vi "parseCameraData.vi"() -> (3 "TargetInfoOut":T1)   [LabVIEW 2012]
uses:
  2013NewCan/Robot Global Data.vi
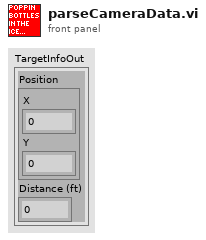
[diagram p1: front panel]
types:
  T1 = cluster{"Position":cluster{"X":dbl, "Y":dbl}, "Distance (ft)":dbl}
  T2 = cluster{"Position":cluster{"X":dbl, "Y":dbl}, "Distance (ft)":dbl}[]
  T3 = cluster{"Target Info[0]":cluster{"Position":cluster{"X":dbl, "Y":dbl}, "Distance (ft)":dbl}, "Target Info[1]":cluster{"Position":cluster{"X":dbl, "Y":dbl}, "Distance (ft)":dbl}, "Target Info[2]":cluster{"Position":cluster{"X":dbl, "Y":dbl}, "Distance (ft)":dbl}, "Target Info[3]":cluster{"Position":cluster{"X":dbl, "Y":dbl}, "Distance (ft)":dbl}, "Target Info[4]":cluster{"Position":cluster{"X":dbl, "Y":dbl}, "Distance (ft)":dbl}, "Target Info[5]":cluster{"Position":cluster{"X":dbl, "Y":dbl}, "Distance (ft)":dbl}, "Target Info[6]":cluster{"Position":cluster{"X":dbl, "Y":dbl}, "Distance (ft)":dbl}, "Target Info[7]":cluster{"Position":cluster{"X":dbl, "Y":dbl}, "Distance (ft)":dbl}, "Target Info[8]":cluster{"Position":cluster{"X":dbl, "Y":dbl}, "Distance (ft)":dbl}}
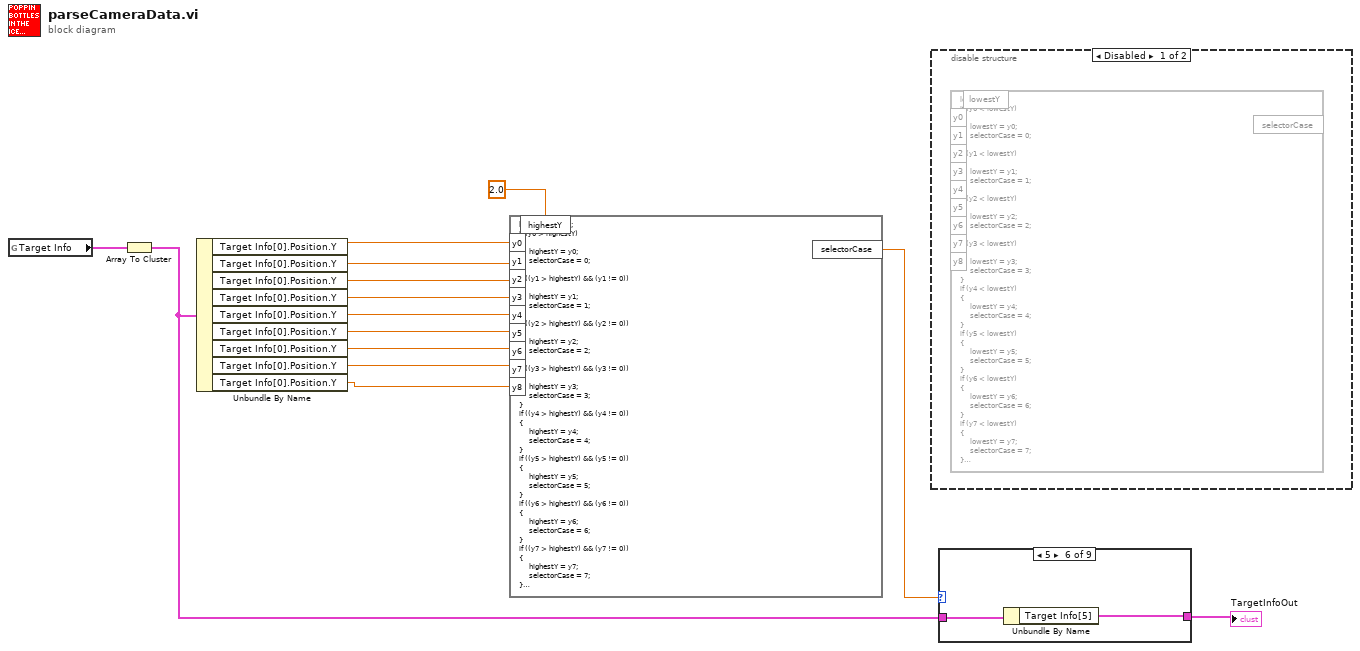
[diagram p0: block diagram]
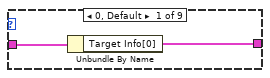
[diagram p3: hidden frame]
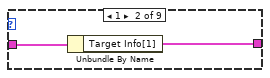
[diagram p4: hidden frame]
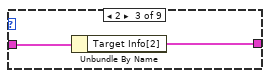
[diagram p5: hidden frame]
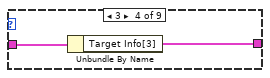
[diagram p6: hidden frame]
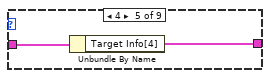
[diagram p7: hidden frame]
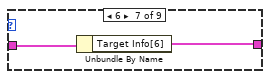
[diagram p8: hidden frame]
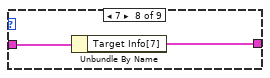
[diagram p9: hidden frame]
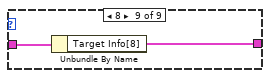
[diagram p10: hidden frame]
diagram:
  n1 = global read "Robot Global Data.vi" "Target Info"() -> (w12:T2)
  n2 = Array To Cluster(array=w12) -> (cluster=w11:T3)
  n3 = Unbundle By Name(w11) -> ("Target Info[0].Position.Y"=w10:dbl, "Target Info[0].Position.Y"=w2:dbl, "Target Info[0].Position.Y"=w3:dbl, "Target Info[0].Position.Y"=w4:dbl, "Target Info[0].Position.Y"=w5:dbl, "Target Info[0].Position.Y"=w6:dbl, "Target Info[0].Position.Y"=w7:dbl, "Target Info[0].Position.Y"=w8:dbl, "Target Info[0].Position.Y"=w9:dbl)
  n4 = formula code="highestY = -2.0;\nif (y0 > highestY)\n{\n     highestY = y0;\n     selectorCase = 0;\n}\nif ((y1 > highestY) && (y1 != 0))\n{\n     highestY = y1;\n     selectorCase = 1;\n}\nif ((y2 > highestY) && (y2 != 0))\n{\n     highestY = y2;\n     selectorCase = 2;\n}\nif ((y3 > highestY) && (y3 != 0))\n{\n     highestY = y3;\n     selectorCase = 3;\n}\nif ((y4 > highestY) && (y4 != 0))\n{\n     highestY = y4;\n     selectorCase = 4;\n}\nif ((y5 > highestY) && (y5 != 0))\n{\n     highestY = y5;\n     selectorCase = 5;\n}\nif ((y6 > highestY) && (y6 != 0))\n{\n     highestY = y6;\n     selectorCase = 6;\n}\nif ((y7 > highestY) && (y7 != 0))\n{\n     highestY = y7;\n     selectorCase = 7;\n}\nif ((y8 > highestY) && (y8 != 0))\n{\n     highestY = y8;\n     selectorCase = 8;\n}"("y0"=w10, "y1"=w2, "y2"=w3, "y3"=w4, "y4"=w5, "y5"=w6, "y6"=w7, "y7"=w8, "y8"=w9, "highestY"=2.0 ("input variable")) -> ("selectorCase"=w13:dbl)
  n5 = disable-structure shown="Disabled" {
    frame Disabled {
      n6 = formula code="lowestY = 2.0;\nif (y0 < lowestY)\n{\n     lowestY = y0;\n     selectorCase = 0;\n}\nif (y1 < lowestY)\n{\n     lowestY = y1;\n     selectorCase = 1;\n}\nif (y2 < lowestY)\n{\n     lowestY = y2;\n     selectorCase = 2;\n}\nif (y3 < lowestY)\n{\n     lowestY = y3;\n     selectorCase = 3;\n}\nif (y4 < lowestY)\n{\n     lowestY = y4;\n     selectorCase = 4;\n}\nif (y5 < lowestY)\n{\n     lowestY = y5;\n     selectorCase = 5;\n}\nif (y6 < lowestY)\n{\n     lowestY = y6;\n     selectorCase = 6;\n}\nif (y7 < lowestY)\n{\n     lowestY = y7;\n     selectorCase = 7;\n}\nif (y8 < lowestY)\n{\n     lowestY = y8;\n     selectorCase = 8;\n}"() -> ()  [unwired: 10 in, 1 out]
    }
    frame Enabled {
    }
  }
  n7 = case shown="5" w13 {
    tunnel: w11 -> [w16 w18 w20 w22 w24 w26 w28 w30 w32]
    tunnel: [w15 w17 w19 w21 w23 w25 w27 w29 w31] -> w1
    frame 0, Default {
      n8 = Unbundle By Name(w16) -> ("Target Info[0]"=w15:T1)
    }
    frame 1 {
      n9 = Unbundle By Name(w18) -> ("Target Info[1]"=w17:T1)
    }
    frame 2 {
      n10 = Unbundle By Name(w20) -> ("Target Info[2]"=w19:T1)
    }
    frame 3 {
      n11 = Unbundle By Name(w22) -> ("Target Info[3]"=w21:T1)
    }
    frame 4 {
      n12 = Unbundle By Name(w24) -> ("Target Info[4]"=w23:T1)
    }
    frame 5 {
      n13 = Unbundle By Name(w26) -> ("Target Info[5]"=w25:T1)
    }
    frame 6 {
      n14 = Unbundle By Name(w28) -> ("Target Info[6]"=w27:T1)
    }
    frame 7 {
      n15 = Unbundle By Name(w30) -> ("Target Info[7]"=w29:T1)
    }
    frame 8 {
      n16 = Unbundle By Name(w32) -> ("Target Info[8]"=w31:T1)
    }
  }
  "TargetInfoOut" <- w1
